vi "Chroma 1905x Series Memory Get Memory Name By Location query.vi"(7 "error in (no error)":errorcluster, 10 "VISA resource name":refnum<visa-resource-name>) -> (0 "error out":errorcluster, 3 "VISA resource name out":refnum<visa-resource-name>, 9 "Name":string)   [LabVIEW 2025]
doc: "Contact Chroma\nTEL: +886-2-2298-3855 \nTEL: +886-3-397-5788 \nFAX: +886-2-2298-3596\nFAX: +886-3-327-4703 \nURL: http://www.chromaate.com \nE-mail: chroma@chroma.com.tw"
uses:
  <instrlib>/Chroma 19052/Chroma 19052.lvlib
panel:
  in  "Memory Location":u32=1 min=1 max=99 step=1
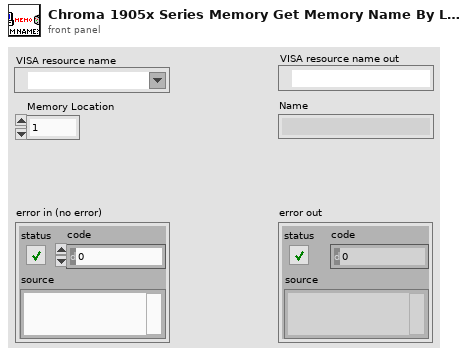
[diagram p1: front panel]
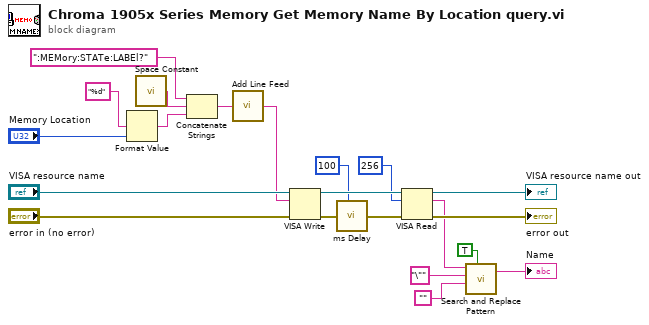
[diagram p0: block diagram]
diagram:
  n1 = Format Value(format string="%d", value (0)="Memory Location") -> (output string=w7:string)  [unwired: 1 in]
  n2 = call <vilib>:"Space Constant.vi"() -> ("String"=w14:string)
  n3 = Concatenate Strings(":MEMory:STATe:LABEl?", w14, w7) -> (w13:string)
  n4 = call <instrlib>:"Add Line Feed.vi"("Command string"=w13) -> ("Concatenated string"=w16:string)  [unwired: 4 in]
  n5 = VISA Write(VISA resource name="VISA resource name", write buffer=w16, error in (no error)="error in (no error)") -> (VISA resource name out=w21:refnum<visa-resource-name>, error out=w11:errorcluster)  [unwired: 1 out]
  n6 = call <instrlib>:"ms Delay.vi"("miliseconds to wait"=u32 100 ("Time Delay ms"), "error in (no error)"=w11) -> ("error out"=w12:errorcluster)  [unwired: 6 in, 1 out]
  n7 = VISA Read(VISA resource name=w21, byte count=u32 256, error in (no error)=w12) -> (VISA resource name out=→"VISA resource name out":refnum<visa-resource-name>, read buffer=w1:string, error out=→"error out":errorcluster)  [unwired: 1 out]
  n8 = call <vilib>:"Search and Replace Pattern.vi"("string"=w1, "regular expression (\"\")"="\"", "replace string (\"\")"="", "replace all? (F)"=TRUE) -> ("result string"=→"Name":string)  [unwired: 1 in, 1 out]
